vi "Read R_W_.vi"(8 "error in (no error)":errorcluster, 11 "BML Pattern Creater in":refnum<class "BML Pattern Creater.lvclass">) -> (0 "error out":errorcluster, 2 "R/W?":T1, 3 "BML Pattern Creater out":refnum<class "BML Pattern Creater.lvclass">)   [LabVIEW 2018, in "BML Pattern Creater.lvlib" / "BML Pattern Creater.lvclass"]
uses:
  BML Pattern Creater.lvclass
  Ctls/RW Options.ctl
  BML Pattern Creater.lvclass/BML Pattern Creater.ctl
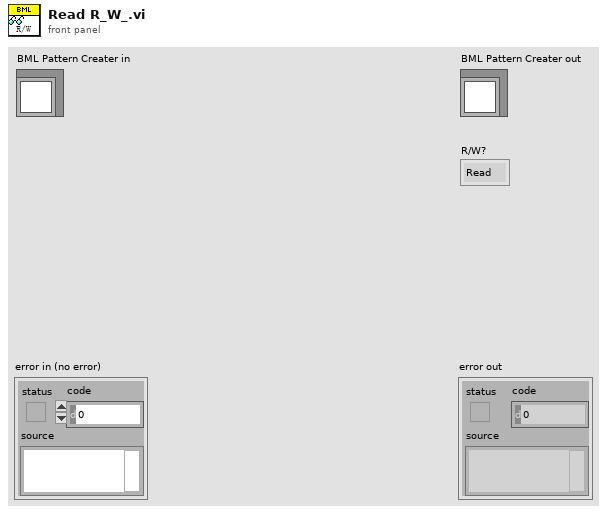
[diagram p1: front panel]
types:
  T1 = typedef "RW Options.ctl" = enum16{"Read", "Write", "R/W"}
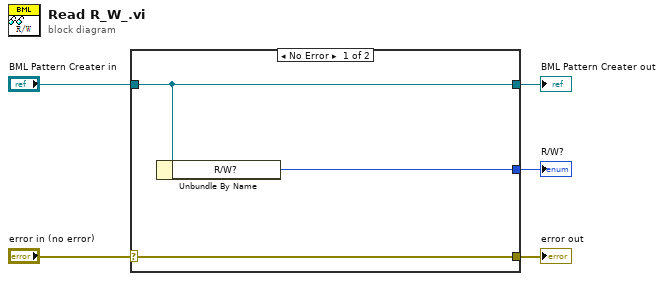
[diagram p0: block diagram]
diagram:
  n1 = case shown="No Error" "error in (no error)" {
    selector: "error in (no error)" -> [w8 w9]
    tunnel: [w8 w9] -> w4
    tunnel: [w7 w10] -> w2
    tunnel: "BML Pattern Creater in" -> [w7 w10]
    tunnel: [w6 _] -> w1
    frame No Error {
      n2 = Unbundle By Name(w7) -> ("R/W?"=w6:T1)
    }
    frame Error {
    }
  }
  "error out" <- w4
  "BML Pattern Creater out" <- w2
  "R/W?" <- w1
